vi "set Misc Info.vi"(8 "error in":errorcluster, 11 "Misc Info":string) -> (0 "error out":errorcluster)   [LabVIEW 2015, in "App Info.lvlib"]
uses:
  App Info.lvlib
  Action.ctl
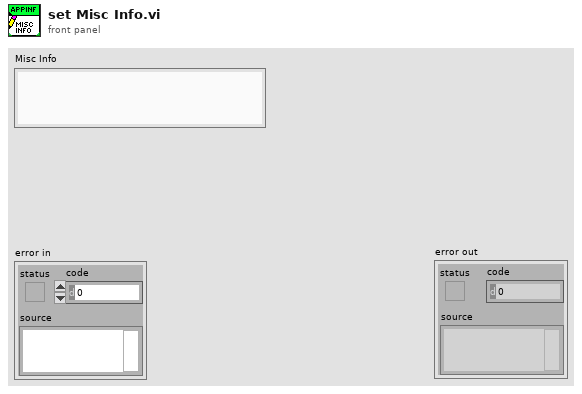
[diagram p1: front panel]
types:
  T1 = typedef "App Info.lvlib/Action.ctl" = enum16{"Initialise", "get All", "set Version", "set Misc Info", "set Name", "set Name 2"}
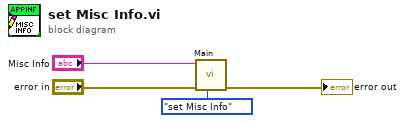
[diagram p0: block diagram]
diagram:
  n1 = call "Main.vi"("Action"=Action."set Misc Info", "error in"="error in", "Data In"="Misc Info") -> ("error out"=→"error out":errorcluster)  [unwired: 7 in, 1 out]
